vi "GetInstrumentInformation.vi"(6 "Timeout(ms)":i32, 8 "error in (no error)":errorcluster, 10 "RoomAlert Device Array Index":i32, 11 "RoomAlert in":refnum<class "RoomAlert.lvclass">) -> (0 "error out":errorcluster, 2 "SNMPDataAsStrings":string[][](array[string]), 3 "RoomAlert out":refnum<class "RoomAlert.lvclass">)   [LabVIEW 2018, in "SensorPlugins.lvlib" / "RoomAlert.lvclass"]
doc: "Extracts the model name of the RoomAlert Instrument and also used to double check the connection to the instrument."
uses:
  RoomAlert.lvclass
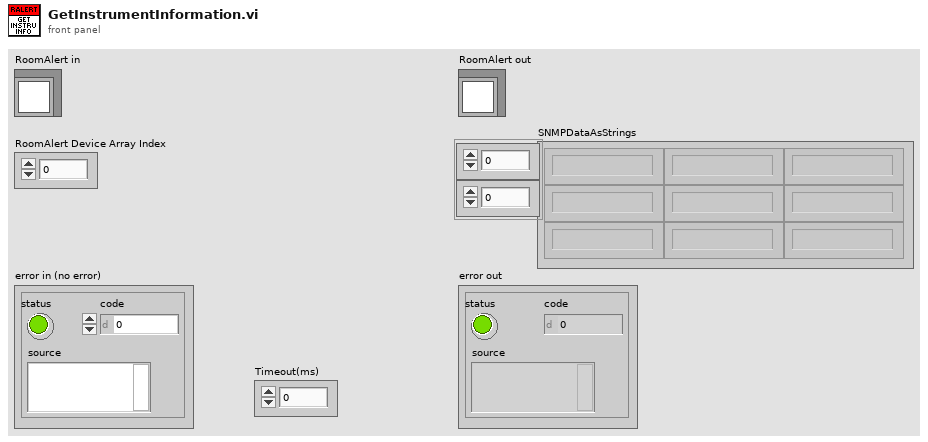
[diagram p1: front panel]
types:
  T1 = typedef "SensorPlugins.lvlib/RoomAlert.lvclass/RoomAlertControls.ctl" = cluster{"Connected?":bool, "IP Address of SNMP Device":string, "Port (161)":u16, "Community Name":string, "Measurements To Read Array":u16[], "Update LightTower?":bool, "LightTower":cluster{"Red":bool, "Amber":bool, "Green":bool, "Audio":bool}, "RoomAlert Model ID":string, "Sensor OID Numbers":string[][], "Sensor Light Tower OID Numbers":string[][]}[]
  T2 = typedef "SensorPlugins.lvlib/RoomAlert.lvclass/CommunicationControls.ctl" = refnum<k16>[]
  T3 = cluster{"Connected?":bool, "IP Address of SNMP Device":string, "Port (161)":u16, "Community Name":string, "Measurements To Read Array":u16[], "Update LightTower?":bool, "LightTower":cluster{"Red":bool, "Amber":bool, "Green":bool, "Audio":bool}, "RoomAlert Model ID":string, "Sensor OID Numbers":string[][], "Sensor Light Tower OID Numbers":string[][]}
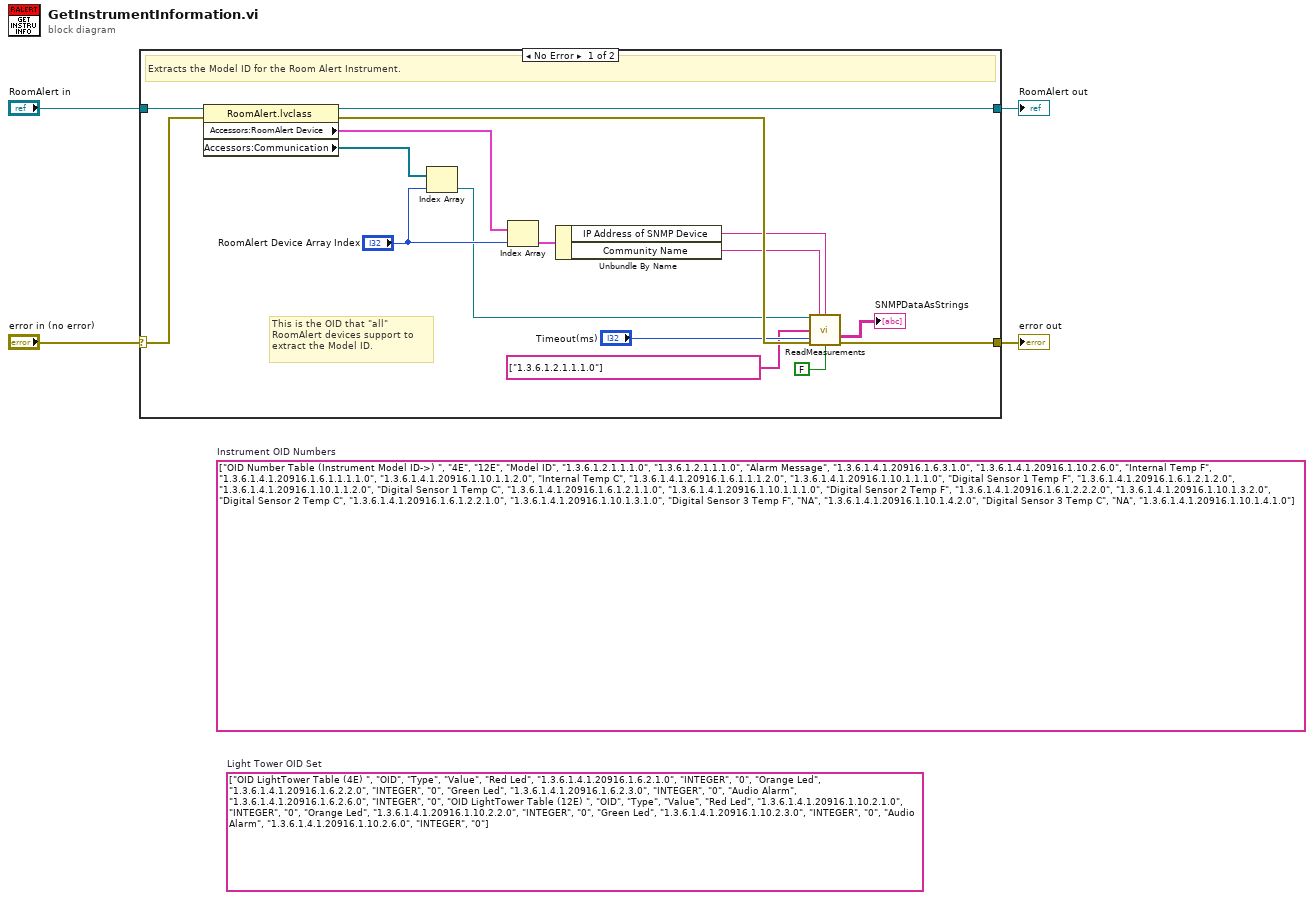
[diagram p0: block diagram]
diagram:
  (unwired) string[][][] [[["OID LightTower Table (4E) ", "OID", "Type", "Value"], ["Red Led", "1.3.6.1.4.1.20916.1.6.2.1.0", "INTEGER", "0"], ["Orange Led", "1.3.6.1.4.1.20916.1.6.2.2.0", "INTEGER", "0"], ["Green Led", "1.3.6.1.4.1.20916.1.6.2.3.0", "INTEGER", "0"], ["Audio Alarm", "1.3.6.1.4.1.20916.1.6.2.6.0", "INTEGER", "0"]], [["OID LightTower Table (12E) ", "OID", "Type", "Value"], ["Red Led", "1.3.6.1.4.1.20916.1.10.2.1.0", "INTEGER", "0"], ["Orange Led", "1.3.6.1.4.1.20916.1.10.2.2.0", "INTEGER", "0"], ["Green Led", "1.3.6.1.4.1.20916.1.10.2.3.0", "INTEGER", "0"], ["Audio Alarm", "1.3.6.1.4.1.20916.1.10.2.6.0", "INTEGER", "0"]]]  # Light Tower OID Set
  (unwired) string[][] [["OID Number Table (Instrument Model ID->) ", "4E", "12E"], ["Model ID", "1.3.6.1.2.1.1.1.0", "1.3.6.1.2.1.1.1.0"], ["Alarm Message", "1.3.6.1.4.1.20916.1.6.3.1.0", "1.3.6.1.4.1.20916.1.10.2.6.0"], ["Internal Temp F", "1.3.6.1.4.1.20916.1.6.1.1.1.1.0", "1.3.6.1.4.1.20916.1.10.1.1.2.0"], ["Internal Temp C", "1.3.6.1.4.1.20916.1.6.1.1.1.2.0", "1.3.6.1.4.1.20916.1.10.1.1.1.0"], ["Digital Sensor 1 Temp F", "1.3.6.1.4.1.20916.1.6.1.2.1.2.0", "1.3.6.1.4.1.20916.1.10.1.1.2.0"], ["Digital Sensor 1 Temp C", "1.3.6.1.4.1.20916.1.6.1.2.1.1.0", "1.3.6.1.4.1.20916.1.10.1.1.1.0"], ["Digital Sensor 2 Temp F", "1.3.6.1.4.1.20916.1.6.1.2.2.2.0", "1.3.6.1.4.1.20916.1.10.1.3.2.0"], ["Digital Sensor 2 Temp C", "1.3.6.1.4.1.20916.1.6.1.2.2.1.0", "1.3.6.1.4.1.20916.1.10.1.3.1.0"], ["Digital Sensor 3 Temp F", "NA", "1.3.6.1.4.1.20916.1.10.1.4.2.0"], ["Digital Sensor 3 Temp C", "NA", "1.3.6.1.4.1.20916.1.10.1.4.1.0"]]  # Instrument OID Numbers
  n1 = case shown="No Error" "error in (no error)" {
    selector: "error in (no error)" -> [w18 w22]
    tunnel: [w17 w22] -> w3
    tunnel: [w19 w21] -> w1
    tunnel: "RoomAlert in" -> [w20 w21]
    frame No Error {
      # "This is the OID that \"all\" \nRoomAlert devices support to \nextract the Model ID."
      # "Extracts the Model ID for the Room Alert Instrument."
      n2 = property class="RoomAlert.lvclass"(reference=w20, error in=w18) -> (reference out=w19:refnum<class "RoomAlert.lvclass">, error out=w15:errorcluster, "Accessors:RoomAlert Device"=w16:T1, "Accessors:Communication "=w11:T2)
      n3 = Index Array(array=w11, index="RoomAlert Device Array Index") -> (element=w9:refnum<k16>)
      n4 = Index Array(array=w16, index="RoomAlert Device Array Index") -> (element=w14:T3)
      n5 = Unbundle By Name(w14) -> ("IP Address of SNMP Device"=w13:string, "Community Name"=w12:string)
      n6 = call "ReadMeasurements.vi"("UDP Network Connection in"=w9, "Community Name"=w12, "IP Address of SNMP Device"=w13, "OID Numbers"=string[] ["1.3.6.1.2.1.1.1.0"], "error in (no error)"=w15, "Timeout(ms)"="Timeout(ms)", "Filter OID Numbers? (T)"=FALSE) -> ("SNMPDataAsStrings"=→"SNMPDataAsStrings":string[][], "error out"=w17:errorcluster)  [unwired: 6 in, 1 out]
    }
    frame Error {
    }
  }
  "error out" <- w3
  "RoomAlert out" <- w1
